vi "Draw Frame.vi"(8 "Error In":errorcluster, 11 "Display Manager In":refnum<class "Display Manager.lvclass">) -> (0 "Error Out":errorcluster, 2 "Frame":u32[][](array[colorbox]), 3 "Display Manager Out":refnum<class "Display Manager.lvclass">)   [LabVIEW 2021, in "Display Manager.lvclass"]
uses:
  Display Manager.lvclass
  Accessors/Display Elements/Get Display Elements.vi
  Accessors/Frame/Get Frame.vi
  Display Element/Display Element.lvclass
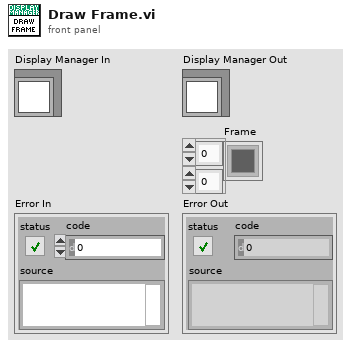
[diagram p1: front panel]
types:
  T1 = typedef "Display Element.lvclass/Pixel.ctl" = cluster{"Position":T2, "Color":u32}
  T2 = typedef "Display Utilities.lvlib/2D Coordinates.ctl" = cluster{"X":i32, "Y":i32}
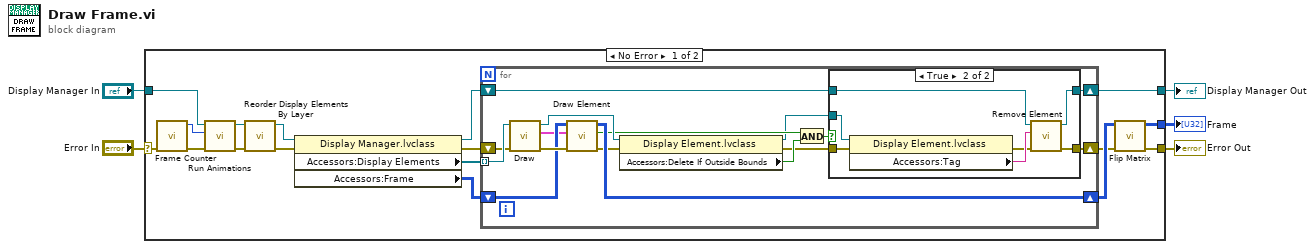
[diagram p0: block diagram]
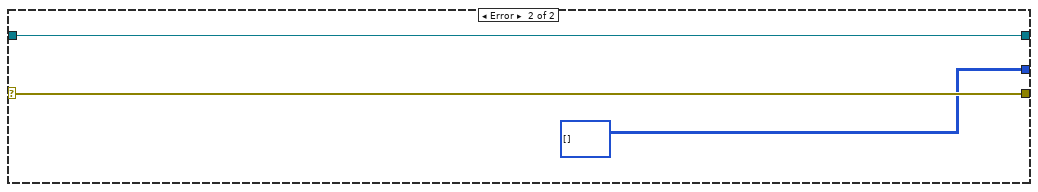
[diagram p3: hidden frame]
diagram:
  n1 = case shown="No Error" "Error In" {
    selector: "Error In" -> [w9 w49]
    tunnel: "Display Manager In" -> [w8 w50]
    tunnel: [w19 w50] -> w3
    tunnel: [w12 w49] -> w2
    tunnel: [w14 u32[][] [] ("Accessors:Frame")] -> w1
    frame No Error {
      n2 = call "Frame Counter.vi"("Error In"=w9) -> ("Error Out"=w7:errorcluster, "Frame Count"=w6:u64)  [unwired: 9 in]
      n3 = call "Run Animations.vi"("Error In"=w7, "Frame Count"=w6, "Display Manager In"=w8) -> ("Error Out"=w10:errorcluster, "Display Manager Out"=w11:refnum<class "Display Manager.lvclass">)  [unwired: 7 in]
      n4 = call "Reorder Display Elements By Layer.vi"("Error In"=w10, "Display Manager In"=w11) -> ("Error Out"=w16:errorcluster, "Display Manager Out"=w17:refnum<class "Display Manager.lvclass">)  [unwired: 8 in]
      n5 = property class="Display Manager.lvclass"(reference=w17, error in=w16) -> (reference out=w20:refnum<class "Display Manager.lvclass">, error out=w21:errorcluster, "Accessors:Display Elements"=w22:refnum<class "Display Element.lvclass">[], "Accessors:Frame"=w18:u32[][])
      n6 = for {
        tunnel: w22 -> [w38] mode=indexing
        shift-right: [w34] -> w13
        shift-left: w21 -> [w37]
        shift-right: [w35] -> w15
        shift-left: w18 -> [w31]
        shift-right: [w32] -> w19
        shift-left: w20 -> [w33]
        n7 = call-dynamic "Draw.vi"("Error In"=w37, "Display Element In"=w38) -> ("Error Out"=w36:errorcluster, "Element To Display"=w30:T1[], "Display Element Out"=w29:refnum<class "Display Element.lvclass">)  [unwired: 7 in]
        n8 = call "Draw Element.vi"("Error In"=w36, "Element To Display"=w30, "Frame In"=w31) -> ("Error Out"=w28:errorcluster, "Frame Changed?"=w27:bool, "Frame Out"=w35:u32[][])  [unwired: 6 in]
        n9 = property class="Display Element.lvclass"(reference=w29, error in=w28) -> (reference out=w25:refnum<class "Display Element.lvclass">, error out=w23:errorcluster, "Accessors:Delete If Outside Bounds"=w26:bool)
        n10 = And(x=w27, y=w26) -> (x .and. y?=w24:bool)
        n11 = case shown="True" w24 {
          tunnel: [w39 w41] -> w34
          tunnel: w33 -> [w40 w47]
          tunnel: [w40 w46] -> w32
          tunnel: w25 -> [_ w45]
          tunnel: w23 -> [w39 w44]
          frame False {
          }
          frame True {
            n12 = property class="Display Element.lvclass"(reference=w45, error in=w44) -> (error out=w42:errorcluster, "Accessors:Tag"=w43:string)  [unwired: 1 out]
            n13 = call "Remove Element.vi"("Error In"=w42, "Element Tag"=w43, "Display Manager In"=w47) -> ("Error Out"=w41:errorcluster, "Display Manager Out"=w46:refnum<class "Display Manager.lvclass">)  [unwired: 7 in]
          }
        }
      }
      n14 = call "Flip Matrix.vi"("Error In"=w13, "Frame In"=w15) -> ("Error Out"=w12:errorcluster, "Frame Out"=w14:u32[][])  [unwired: 8 in]
    }
    frame Error {
    }
  }
  "Display Manager Out" <- w3
  "Error Out" <- w2
  "Frame" <- w1
